vi "get_Component.vi"(0 "HGF_Composite":refnum<class "HGF_Composite.lvclass">, 2 "objectName":string, 3 "objectIndex":i32, 5 "error in (no error)":errorcluster) -> (14 "dup HGF_Composite":refnum<class "HGF_Composite.lvclass">, 16 "HGF_Component":refnum<class "HGF_Component.lvclass">, 19 "error out":errorcluster)   [LabVIEW 2014, in "HGF_BaseClasses.lvlib" / "HGF_Composite.lvclass"]
doc: "Get a copy of a Component object from Composite object.\n\nYou can specify either objectName or objectIndex.\nIf objectName is empty string the objectIndex will be used."
uses:
  HGF_Composite.lvclass
  HGF_Component/HGF_Component.lvclass
  HGF_Factory/HGF_Factory.lvclass
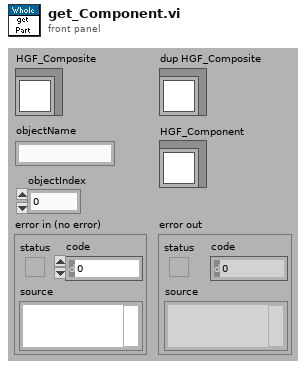
[diagram p1: front panel]
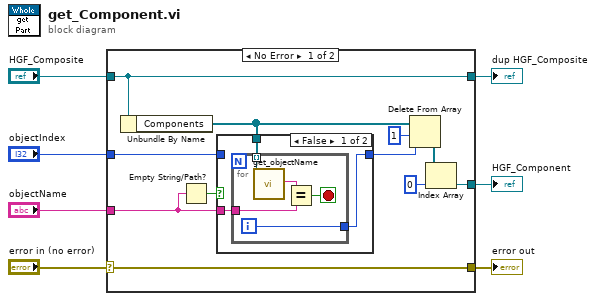
[diagram p0: block diagram]
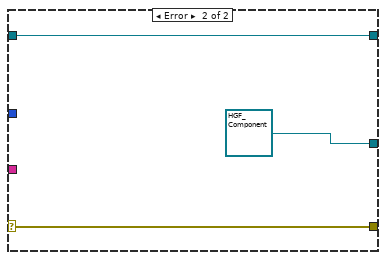
[diagram p3: hidden frame]
diagram:
  n1 = case shown="No Error" "error in (no error)" {
    selector: "error in (no error)" -> [w18 w30]
    tunnel: [w18 w30] -> w6
    tunnel: [w8 w29] -> w4
    tunnel: "HGF_Composite" -> [w8 w29]
    tunnel: "objectIndex" -> [w11 _]
    tunnel: [w14 refnum<class "HGF_Component.lvclass"> refnum ("HGF_Component.lvclass")] -> w2
    tunnel: "objectName" -> [w9 _]
    frame No Error {
      n2 = Unbundle By Name(w8) -> ("Components"=w13:refnum<class "HGF_Component.lvclass">[])
      n3 = Empty String/Path?(string/path=w9) -> (empty?=w10:bool)
      n4 = case shown="False" w10 {
        tunnel: w13 -> [w21 _]
        tunnel: w9 -> [w20 _]
        tunnel: [w19 w27] -> w12
        tunnel: w11 -> [_ w27]
        frame False {
          n5 = for {
            tunnel: w21 -> [w26] mode=indexing
            tunnel: w20 -> [w23]
            tunnel: [w22] -> w19
            i -> [w22]
            stop <- w25 stop-if-true
            n6 = call "get_objectName.vi"("HGF_Factory"=w26) -> ("objectName"=w24:string)  [unwired: 1 in, 17 out]
            n7 = Equal?(x=w24, y=w23) -> (x = y?=w25:bool)
          }
        }
        frame True {
        }
      }
      n8 = Delete From Array(array=w13, length=1, index=w12) -> (deleted portion=w17:refnum<class "HGF_Component.lvclass">[])  [unwired: 1 out]
      n9 = Index Array(array=w17, index=0) -> (element=w14:refnum<class "HGF_Component.lvclass">)
    }
    frame Error {
    }
  }
  "error out" <- w6
  "dup HGF_Composite" <- w4
  "HGF_Component" <- w2
